vi "Dequeue Message.vi"(8 "error in":errorcluster, 11 "Module Data In":refnum<class "Rename.lvclass">) -> (0 "error out":errorcluster, 1 "Module Action":string, 2 "Message Data":variant, 3 "Module Data Out":refnum<class "Rename.lvclass">, 4 "Acknowledge Data":T1)   [LabVIEW 2015, in "Generic Module Library.lvlib" / "Template G_Module.lvlib"]
uses:
  Template G_Module.lvlib
  Module Communications/Queue Support/Queue Reference Actions.ctl
  Module Class/Rename.lvclass
  Private Controls/Module Message Cluster Components/Acknowledge Data Cluster.ctl
  Private Controls/Module Message Cluster Components/Ack Payload.ctl
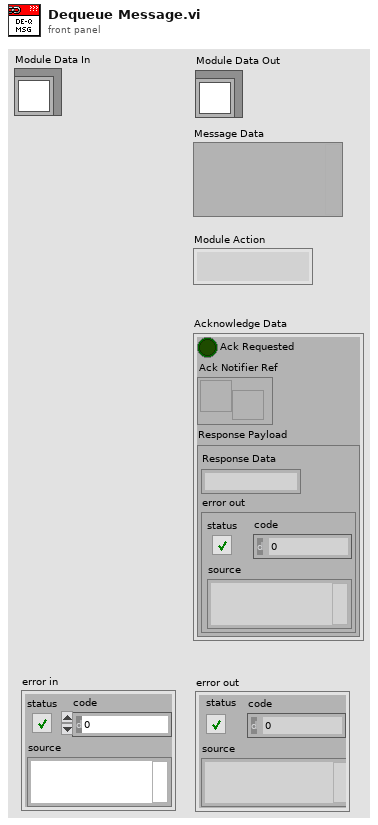
[diagram p1: front panel]
types:
  T1 = typedef "Generic Module Library.lvlib/Template G_Module.lvlib/Acknowledge Data Cluster.ctl" = cluster{"Ack Requested":bool, "Ack Notifier Ref":refnum<notifier>, "Response Payload":T2}
  T2 = typedef "Generic Module Library.lvlib/Template G_Module.lvlib/Ack Payload.ctl" = cluster{"Response Data":string, "error out":errorcluster}
  T3 = typedef "Generic Module Library.lvlib/Template G_Module.lvlib/Queue Reference Actions.ctl" = enum16{"Release", "Set", "Get"}
  T4 = typedef "Generic Module Library.lvlib/Template G_Module.lvlib/Module Message Cluster.ctl" = cluster{"Message Data":T5, "Acknowledge Data":T1}
  T5 = typedef "Generic Module Library.lvlib/Template G_Module.lvlib/Message Data Cluster.ctl" = cluster{"Module Action":string, "Message Data":variant}
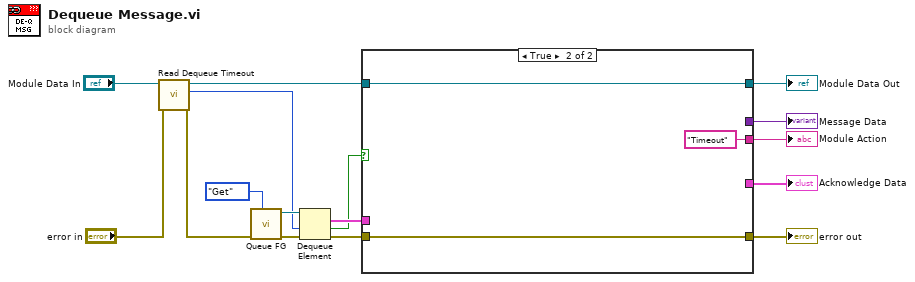
[diagram p0: block diagram]
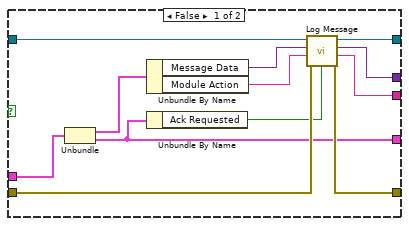
[diagram p2: hidden frame]
diagram:
  n1 = call-dynamic "Read Dequeue Timeout.vi"("error in (no error)"="error in", "Rename in"="Module Data In") -> ("error out"=w2:errorcluster, "Dequeue Timeout"=w1:i32, "Rename out"=w4:refnum<class "Rename.lvclass">)  [unwired: 7 in]
  n2 = call "Queue FG.vi"("Queue Reference Actions"=Queue_Reference_Actions."Get", "error in"=w2) -> ("error out"=w15:errorcluster, "Queue out"=w14:refnum<queue>)  [unwired: 8 in]
  n3 = Dequeue Element(queue=w14, timeout in ms (-1)=w1, error in (no error)=w15) -> (element=w13:T4, timed out?=w6:bool, error out=w11:errorcluster)  [unwired: 1 out]
  n4 = case shown="True" w6 {
    tunnel: w13 -> [w28 _]
    tunnel: w4 -> [w26 w31]
    tunnel: [w25 w31] -> w12
    tunnel: w11 -> [w24 w29]
    tunnel: [w23 w29] -> w10
    tunnel: [w20 "Timeout" ("Module Action")] -> w9
    tunnel: [w19 _] -> w8
    tunnel: [w18 _] -> w7
    frame False {
      n5 = Unbundle(w28) -> ("Message Data"=w27:T5, "Acknowledge Data"=w18:T1)
      n6 = Unbundle By Name(w27) -> ("Message Data"=w22:variant, "Module Action"=w21:string)
      n7 = Unbundle By Name(w18) -> ("Ack Requested"=w17:bool)
      n8 = call "Log Message.vi"("Ack Requested"=w17, "error in"=w24, "Module Action"=w21, "Message Data In"=w22, "Module Data In"=w26) -> ("error out"=w23:errorcluster, "Module Action"=w20:string, "Message Data Out"=w19:variant, "Module Data Out"=w25:refnum<class "Rename.lvclass">)  [unwired: 3 in]
    }
    frame True {
    }
  }
  "error out" <- w10
  "Message Data" <- w8
  "Module Action" <- w9
  "Module Data Out" <- w12
  "Acknowledge Data" <- w7
